vi "Modbus Display Time Real Time Clock.vi"(10 "Absolute Time":dbl, 11 "Timing in in":T1 {"Absolute Time" format="%<%H:%M:%S%3u>t"; "Display Time" format="%#.20f"; "Test Time Ref" format="%#.20f"; "Precondition Time Ref" format="%#.20f"; "First Call Time Ref" format="%#.20f"}) -> (3 "Timing out":T1 {"Absolute Time" format="%<%H:%M:%S%3u>t"; "Display Time" format="%#.20f"; "Test Time Ref" format="%#.20f"; "Precondition Time Ref" format="%#.20f"; "First Call Time Ref" format="%#.20f"})   [LabVIEW 2020, in "Modbus.lvlib"]
uses:
  Modbus.lvlib
  Modbus Timing.ctl
  <vilib>/Utility/miscctls.llb/LVDateTimeRec.ctl
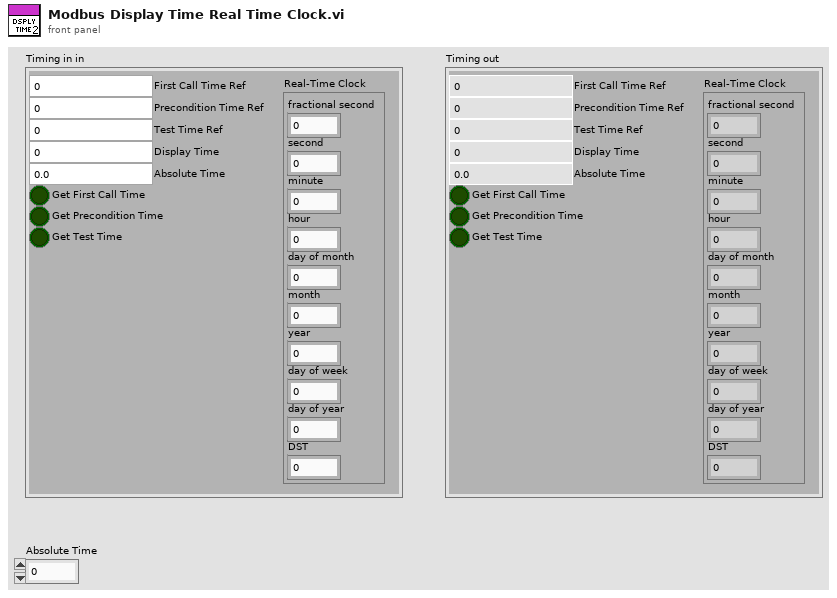
[diagram p1: front panel]
types:
  T1 = typedef "Modbus Timing.ctl" = cluster{"First Call Time Ref":dbl, "Precondition Time Ref":dbl, "Test Time Ref":dbl, "Get First Call Time":bool, "Get Precondition Time":bool, "Get Test Time":bool, "Display Time":dbl, "Real-Time Clock":T2, "Absolute Time":dbl}
  T2 = typedef "LVDateTimeRec.ctl" = cluster{"fractional second":dbl, "second":i32, "minute":i32, "hour":i32, "day of month":i32, "month":i32, "year":i32, "day of week":i32, "day of year":i32, "DST":i32}
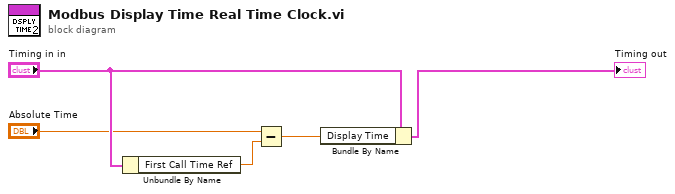
[diagram p0: block diagram]
diagram:
  n1 = Unbundle By Name("Timing in in") -> ("First Call Time Ref"=w2:dbl)
  n2 = Subtract(x="Absolute Time", y=w2) -> (x-y=w5:dbl)
  n3 = Bundle By Name(cluster="Timing in in", "Display Time"=w5) -> (→"Timing out":T1)
